vi "Cam start task.vi"(8 "error in (no error)":errorcluster, 11 "Camera in":refnum<class "Camera.lvclass">) -> (0 "error out":errorcluster, 3 "Camera out":refnum<class "Camera.lvclass">)   [LabVIEW 2021, in "Camera.lvlib" / "Camera.lvclass"]
uses:
  Camera.lvclass
  C:/Program Files (x86)/National Instruments/LabVIEW 2021/vi.lib/ActorFramework/Actor/Actor.lvclass
  Camera.lvclass/Camera.ctl
  Main_Control/Main_Control/notifications.ctl
  <vilib>/ActorFramework/Actor/Actor.lvclass/Actor.ctl
  Main_Control/Main_Control Messages/UI notifier Msg/UI notifier Msg.lvclass/UI notifier Msg.ctl
  <vilib>/ActorFramework/Message Enqueuer/Message Enqueuer.lvclass/Message Enqueuer.ctl
  <vilib>/ActorFramework/Message Enqueuer/Enqueue.vi
  Main_Control/Main_Control Messages/UI notifier Msg/UI notifier Msg.lvclass
  C:/Program Files (x86)/National Instruments/LabVIEW 2021/vi.lib/ActorFramework/Message/Message.lvclass
  <vilib>/ActorFramework/Message Priority Queue/Priority Enqueue.vi
  <vilib>/ActorFramework/Actor/Actor.lvclass
  Main_Control/Main_Control/Main_Control.lvclass
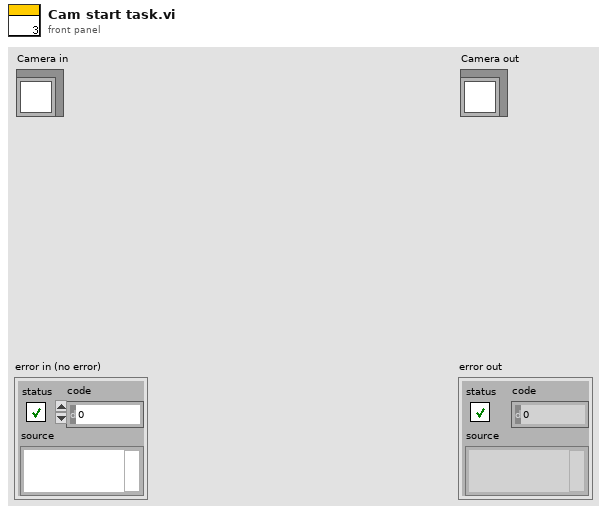
[diagram p1: front panel]
types:
  T1 = typedef "Main_Control.lvlib/Main_Control.lvclass/notifications.ctl" = enum16{"cam 1 frame skkipped", "cam finish", "cam started", "cam stopped", "cam updated", "ni started", "ni stopped", "ni updated"}
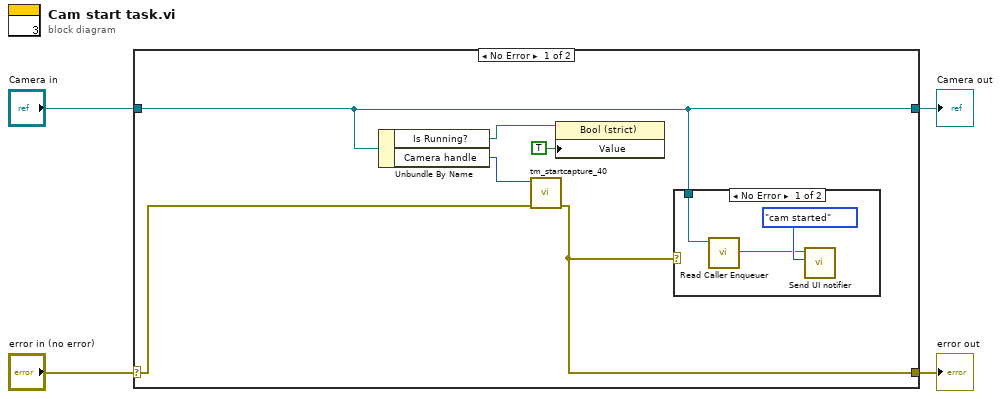
[diagram p0: block diagram]
diagram:
  n1 = case shown="No Error" "error in (no error)" {
    selector: "error in (no error)" -> [w5 w15]
    tunnel: [w7 w15] -> w3
    tunnel: [w6 w14] -> w1
    tunnel: "Camera in" -> [w6 w14]
    frame No Error {
      n2 = Unbundle By Name(w6) -> ("Is Running?"=w9:refnum<vi>, "Camera handle"=w10:u32)
      n3 = call <userlib>:"tm_startcapture_40.vi"("error in (no error)"=w5, "Handle in"=w10) -> ("error out"=w7:errorcluster)  [unwired: 8 in, 1 out]
      n4 = property class="Bool (strict)"(reference=w9, "Value"=TRUE) -> ()  [unwired: 1 in, 2 out]
      n5 = case shown="No Error" w7 {
        tunnel: w6 -> [w13 _]
        frame No Error {
          n6 = call <vilib>:"Read Caller Enqueuer.vi"("Actor"=w13) -> ("Caller Enqueuer"=w11:refnum<class "Message Enqueuer.lvclass">)  [unwired: 10 in]
          n7 = call "Send UI notifier.vi"("Object&State"=notifications."cam started", "Message Enqueuer"=w11) -> ()  [unwired: 8 in, 2 out]
        }
        frame Error {
        }
      }
    }
    frame Error {
    }
  }
  "error out" <- w3
  "Camera out" <- w1
